vi "Calc_rhozero.vi"(0 "Q":dbl[](array[numeric])) -> (7 "rho+":dbl[](array[numeric]))   [LabVIEW 2018]
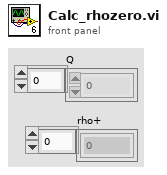
[diagram p1: front panel]
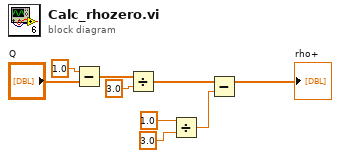
[diagram p0: block diagram]
diagram:
  n1 = Subtract(x=1.0, y="Q") -> (x-y=w6:dbl[])
  n2 = Divide(x=w6, y=3.0) -> (x/y=w5:dbl[])
  n3 = Divide(x=1.0, y=3.0) -> (x/y=w1:dbl)
  n4 = Subtract(x=w5, y=w1) -> (x-y=→"rho+":dbl[])
